vi "DSF.Shared.Data Type.Sizeof.vi"(11 "data type":T1) -> (2 "bitshift count":u8, 3 "size in bytes":u64 format="%d bytes")   [LabVIEW 2017, in "Data Sharing Framework Engine.lvlib"]
uses:
  Source/Data Sharing Framework Core/Engine/Data Sharing Framework Engine.lvlib
  DSF Configuration API/1.0.0/Public/Controls/DSF Data Type.ctl
  DSF Configuration API/1.0.0/DSF Configuration API.lvlib
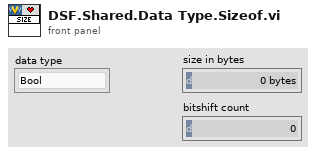
[diagram p1: front panel]
types:
  T1 = typedef "DSF Configuration API.lvlib/DSF Data Type.ctl" = enum8{"Bool", "SGL", "DBL", "I8", "I16", "I32", "I64", "U8", "U16", "U32", "U64"}
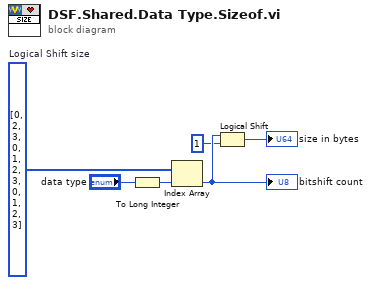
[diagram p0: block diagram]
diagram:
  w6 = u8[] [0, 2, 3, 0, 1, 2, 3, 0, 1, 2, 3]  # Logical Shift size
  n1 = To Long Integer(number="data type") -> (32bit integer=w5:i32)
  n2 = Index Array(array=w6, index=w5) -> (element=w4:u8)
  "bitshift count" <- w4
  n3 = Logical Shift(y=w4, x=u64 1) -> (x << y=→"size in bytes":u64)
